vi "Autonomous Independent.vi"() -> ()   [LabVIEW 2016]
doc: "This VI is called when autonomous begins, and will automatically be terminated when autonomous ends. You can carry out timed or sensor driven robot movement independently without needing to return to the caller."
uses:
  <vilib>/Rock Robotics/WPI/Utilities/WPI_GetSetVariantRefNum.vi
  <vilib>/Rock Robotics/Network Tables/NT Write Numeric Array.vi
  Alliance_ID.vi
  <vilib>/Rock Robotics/WPI/RobotDrive/WPI_RobotDriveArcadeDrive_Standard(NoSaturation).vi
  <vilib>/Rock Robotics/Network Tables/NT Read String.vi
  <vilib>/Rock Robotics/Network Tables/NT Write Number.vi
panel:
  out "Completed Task 8":bool
  in  "Past the Peg. No Turn":i32=18
  out "Completed Task 7":bool
  in  "Ticks to the Peg 6":i32=3
  in  "Ticks to the Peg 5":i32=19
  out "Count":dbl
  in  "Ticks to the Peg 4":i32=3
  out "Completed Task 6":bool
  out "Completed Task 5":bool
  out "Completed Task 4":bool
  out "Completed Task 3":bool
  in  "Ticks to the Peg 3":i32=20
  out "Completed Task 1":bool
  in  "Ticks to the Peg 2":i32=15
  out "Left + Right OverSpeed":cluster{dbl, dbl}(knob)={10.0, -10.0} scale=-10.0..10.0
  out "Difference":dbl(knob) scale=0.0..50.0
  out "Right Wheel Sensor Count":dbl
  out "Left Wheel Sensor Count":dbl
  in  "Reset Counters":bool
  # "ALT 1"
  # "Position 3"
  # "16"
  # "20"
  # "Forward"
  # "3"
  # "Foward to the Left"
  # "4"
  # "Position 1"
  # "20"
  # "Forward"
  # "3"
  # "Foward to the Right"
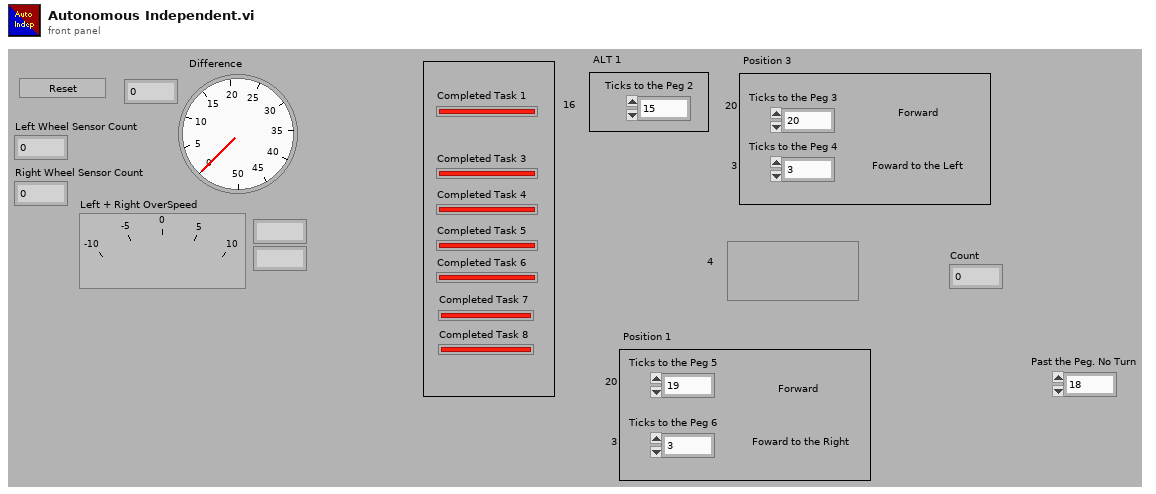
[diagram p1: front panel]
types:
  T1 = typedef "WPI_DriverStationPositionInfo.ctl" = enum16{"1", "2", "3"}
  T2 = typedef "WPI_DriverStationAllianceInfo.ctl" = enum16{"Red", "Blue", "Invalid"}
  T3 = typedef "WPI_JoystickDevRef.ctl" = cluster{"Device":T4}
  T4 = typedef "WPI_JoystickDeviceEnum.ctl" = enum16{"USB 0", "USB 1", "USB 2", "USB 3", "USB 4", "USB 5"}
  T5 = typedef "WPI_RobotDriveDevRef.ctl" = cluster{"DevStatus":errorcluster, "Motors[]":T6[], "Square Inputs":bool, "Max Output":dbl}
  T6 = typedef "WPI_MotorControlDeviceRef.ctl" = cluster{"DeviceStatus":errorcluster, "Type":T7, "PWM":cluster{"PWM Channel":T8, "DeadBand":T9}, "CAN":cluster{"Device Number":u8, "SetOutput VI Ref":variant, "GetOutput VI Ref":variant, "Enable VI Ref":variant, "Disable VI Ref":variant, "Data":variant}, "Invert":bool}
  T7 = typedef "WPI_MotorControlType.ctl" = enum16{"PWM", "CAN"}
  T8 = typedef "FPGA_DIOPWMChannel.ctl" = enum8{"PWM 0", "PWM 1", "PWM 2", "PWM 3", "PWM 4", "PWM 5", "PWM 6", "PWM 7", "PWM 8", "PWM 9", "PWM MXP 0", "PWM MXP 1", "PWM MXP 2", "PWM MXP 3", "PWM MXP 4", "PWM MXP 5", "PWM MXP 6", "PWM MXP 7", "PWM MXP 8", "PWM MXP 9", "Invalid"}
  T9 = typedef "WPI_PWMDeadband.ctl" = cluster{"Name":string, "maxPositivePwm":i32, "minPositivePwm":i32, "centerPwm":i32, "maxNegativePwm":i32, "minNegativePwm":i32, "angularRange":u16}
  T10 = typedef "WPI_CounterDevRef.ctl" = cluster{"DevStatus":errorcluster, "CntIndex":T11}
  T11 = typedef "FPGA_CounterCtrSystemIndex.ctl" = enum8{"Ctr 0", "Ctr 1", "Ctr 2", "Ctr 3", "Ctr 4", "Ctr 5", "Ctr 6", "Ctr 7", "Invalid"}
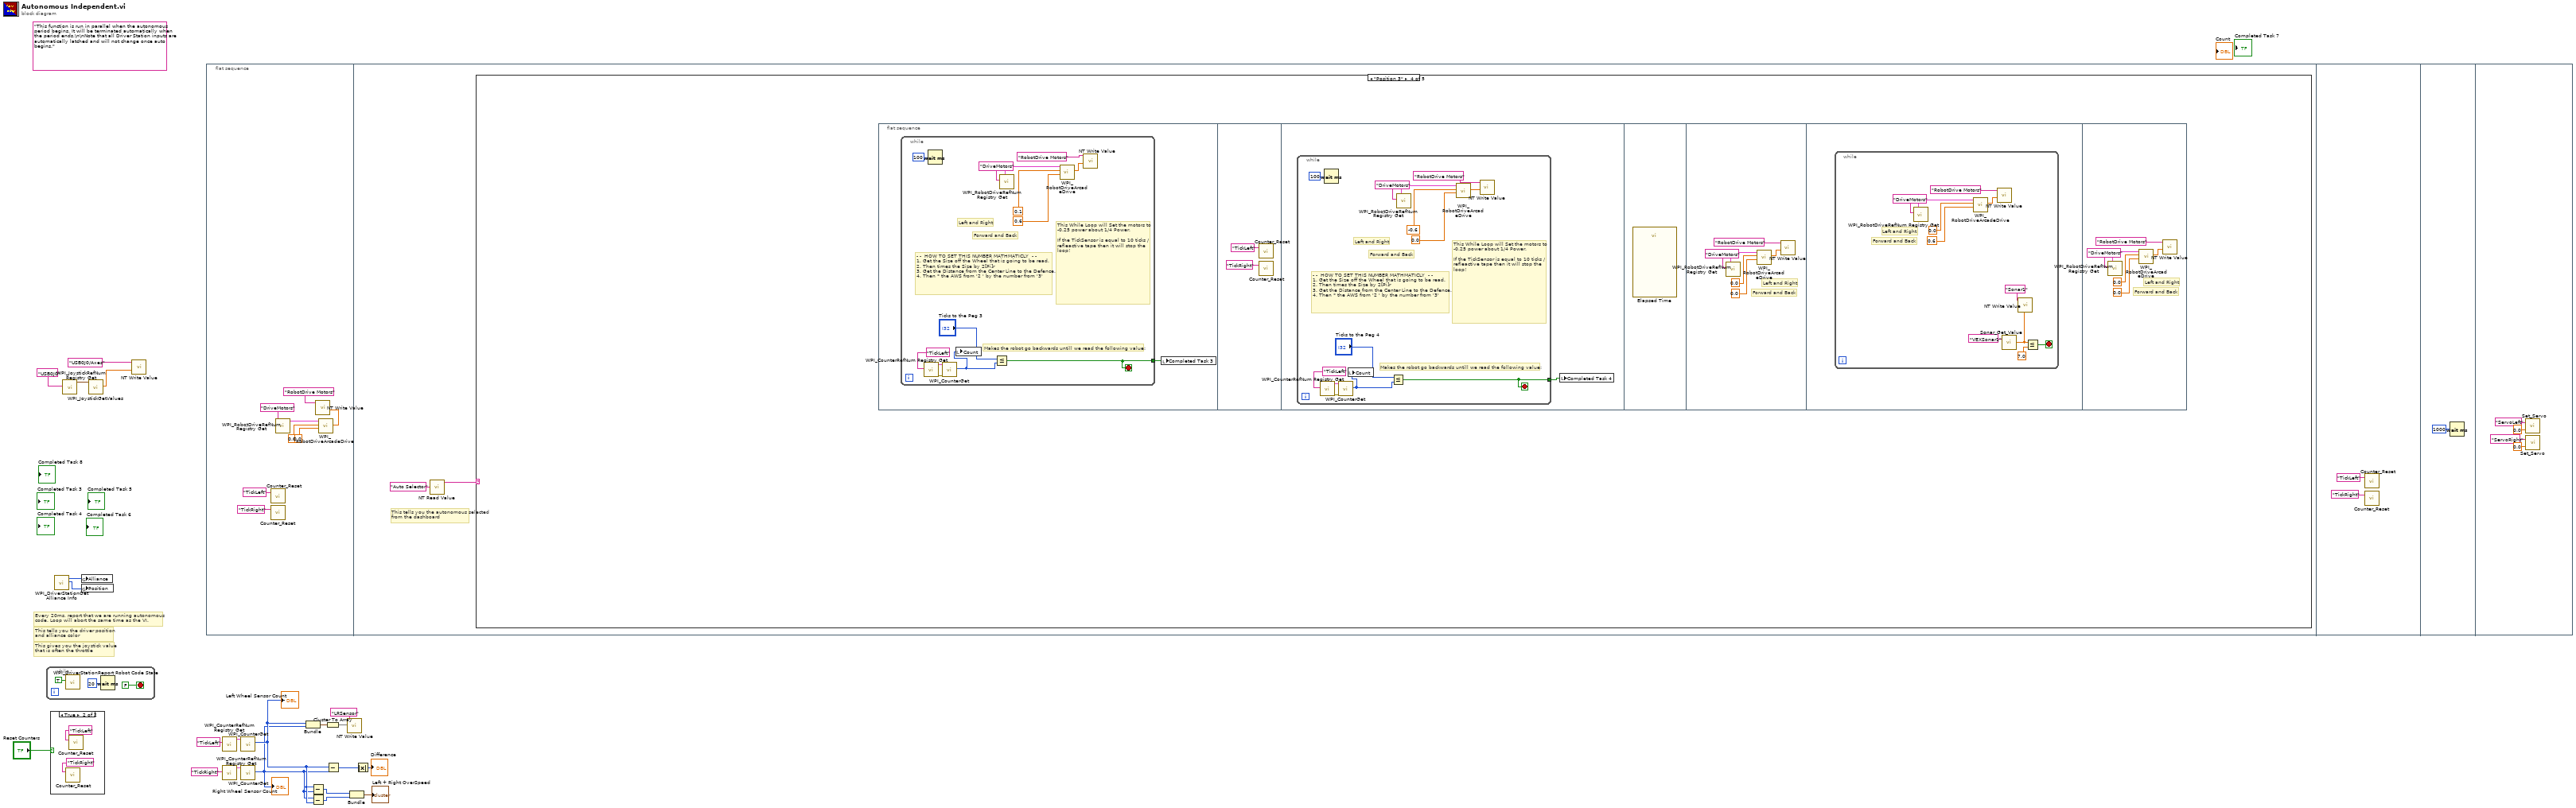
[diagram p0: block diagram]
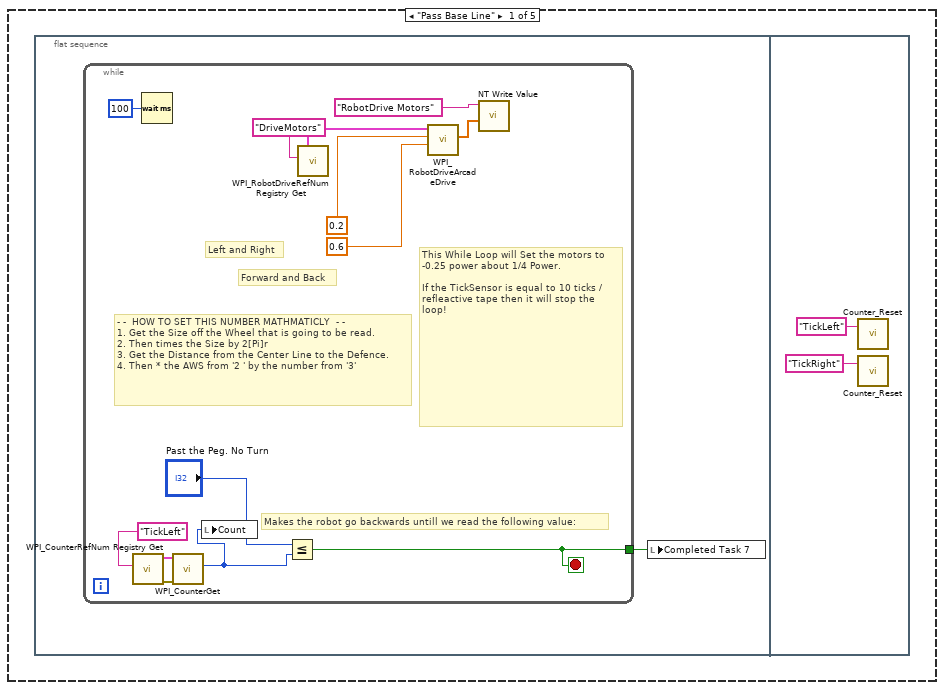
[diagram p2: hidden frame]
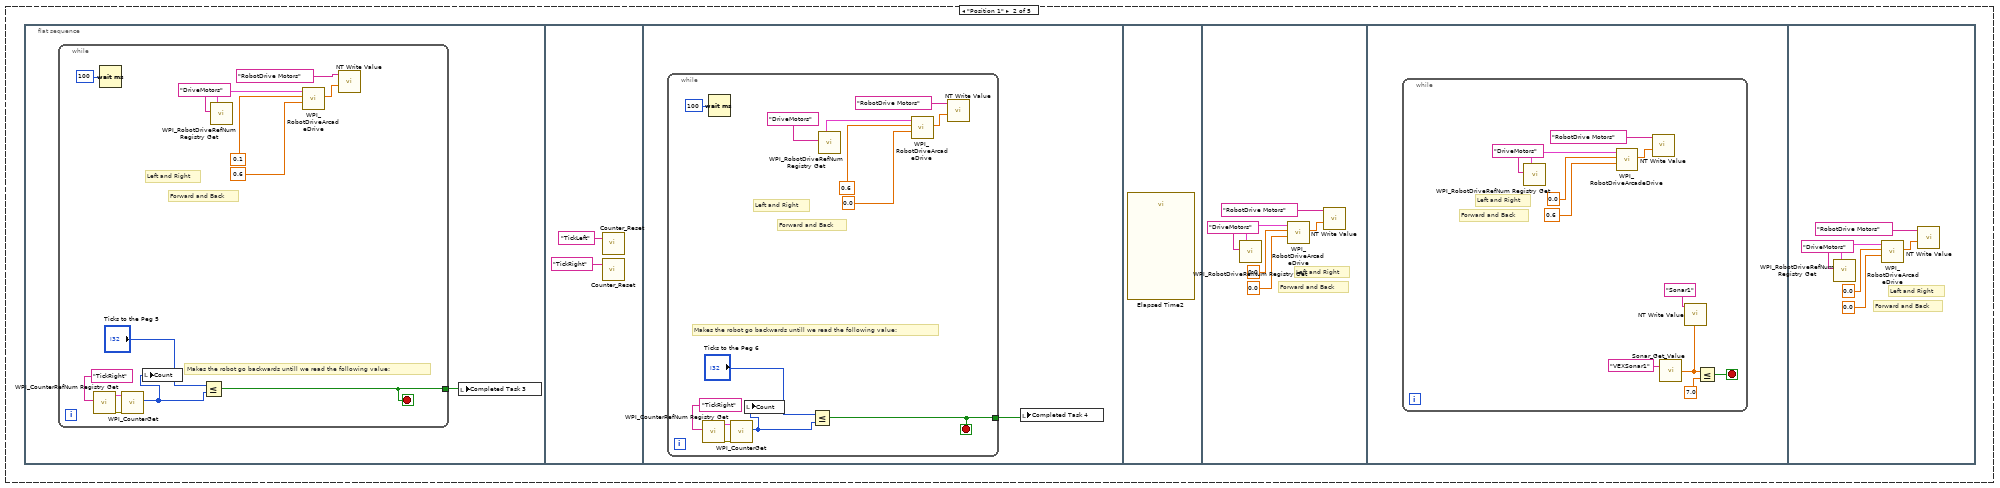
[diagram p3: hidden frame]
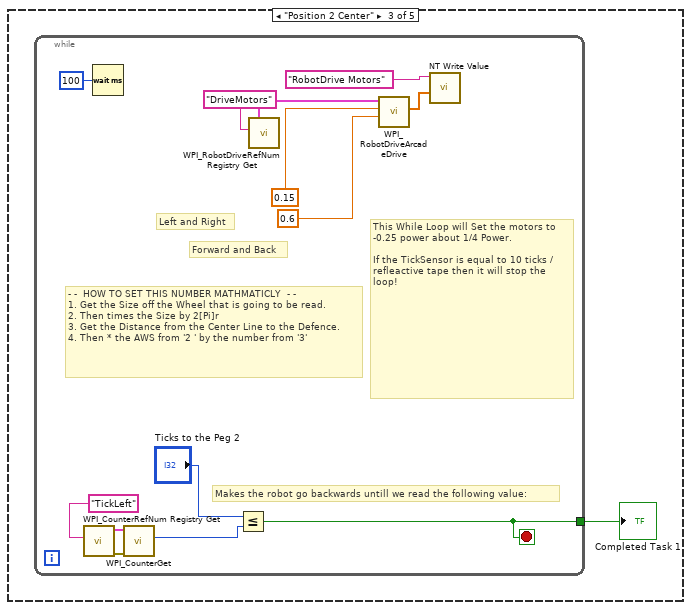
[diagram p4: hidden frame]
diagram:
  (unwired) "This function is run in parallel when the autonomous period begins. It will be terminated automatically when the period ends.\n\nNote that all Driver Station inputs are automatically latched and will not change once auto begins."
  # "Every 20ms, report that we are running autonomous\ncode. Loop will abort the same time as the VI."
  # "This gives you the joystick value\nthat is often the throttle"
  # "This tells you the driver position\nand alliance color"
  n1 = while {
    stop <- FALSE stop-if-true
    n2 = call <vilib>:"WPI_DriverStationReport Robot Code State.vi"("Autonomous"=TRUE) -> ()  [unwired: 10 in, 1 out]
    n3 = Wait (ms)(milliseconds to wait=u32 20) -> ()  [unwired: 1 out]
  }
  n4 = case shown="True" "Reset Counters" {
    frame False {
      # "Do nothing."
    }
    frame True {
      n5 = call "Counter_Reset.vi"("Control"="TickRight" ("refnum name")) -> ()  [unwired: 1 in, 2 out]
      n6 = call "Counter_Reset.vi"("Control"="TickLeft" ("refnum name")) -> ()  [unwired: 1 in, 2 out]
    }
  }
  n7 = call <vilib>:"WPI_DriverStationGet Alliance Info.vi"() -> ("Position"=w6:T1, "Alliance"=w7:T2)  [unwired: 10 out]
  n8 = call <vilib>:"WPI_JoystickRefNum Registry Get.vi"("refnum name"="USB0J0") -> ("JoystickDevRef"=w20:T3)  [unwired: 1 in, 9 out]
  n9 = global write "Alliance_ID.vi" "Alliance"(w7) -> ()
  n10 = global write "Alliance_ID.vi" "Position"(w6) -> ()
  n11 = call <vilib>:"WPI_JoystickGetValues.vi"("JoystickDevRef"=w20) -> ("Axes"=w18:dbl[])  [unwired: 6 in, 4 out]
  n12 = call-poly <vilib>:"NT Write Value.vi"("Numeric Array"=w18, "Name"="USB0J0/Axes") -> ()  [unwired: 9 in, 1 out]
  n13 = flat-sequence {
    frame #0 {
      n14 = call "Counter_Reset.vi"("Control"="TickLeft" ("refnum name")) -> ()  [unwired: 1 in, 2 out]
      n15 = call "Counter_Reset.vi"("Control"="TickRight" ("refnum name")) -> ()  [unwired: 1 in, 2 out]
      n16 = call <vilib>:"WPI_RobotDriveRefNum Registry Get.vi"("refnum name"="DriveMotors") -> ("RobotDriveDevRef"=w34:T5)  [unwired: 1 in, 9 out]
      n17 = call-poly <vilib>:"WPI_RobotDriveArcadeDrive.vi"("Y axis value"=0.0 ("X axis value"), "X axis value"=0.0, "RobotDriveDevRef"=w34) -> ("Motor Values"=w32:dbl[])  [unwired: 1 in, 7 out]
      n18 = call-poly <vilib>:"NT Write Value.vi"("Numeric Array"=w32, "Name"="RobotDrive Motors") -> ()  [unwired: 9 in, 1 out]
    }
    frame #1 {
      # "This tells you the autonomous selected\nfrom the dashboard"
      n19 = call-poly <vilib>:"NT Read Value.vi"("Name"="Auto Selector") -> ("String"=w35:string)  [unwired: 9 in, 1 out]
      n20 = case shown="\"Position 3\"" w35 {
        frame "Pass Base Line" {
          n21 = flat-sequence {
            frame #0 {
              n22 = while {
                tunnel: [w40] -> w37
                stop <- w40 stop-if-true
                # "- -  HOW TO SET THIS NUMBER MATHMATICLY  - - \n1. Get the Size off the Wheel that is going to be read.\n2. Then times the Size by 2[Pi]r\n3. Get the Distance from the Center Line to the Defence.\n4. Then * the AWS from '2 ' by the number from '3'"
                # "Makes the robot go backwards untill we read the following value:"
                # "This While Loop will Set the motors to -0.25 power about 1/4 Power.\n\nIf the TickSensor is equal to 10 ticks / refleactive tape then it will stop the loop!"
                # "Forward and Back"
                # "Left and Right"
                n23 = call <vilib>:"WPI_CounterRefNum Registry Get.vi"("refnum name"="TickLeft") -> ("error out"=w49:errorcluster, "CounterDevRef"=w48:T10)  [unwired: 9 in]
                n24 = Wait (ms)(milliseconds to wait=u32 100) -> ()  [unwired: 1 out]
                n25 = call <vilib>:"WPI_CounterGet.vi"("error in (no error)"=w49, "CounterDevRef in"=w48) -> ("Value"=w38:i32)  [unwired: 4 in, 5 out]
                n26 = local write "Count"(w38) -> ()
                n27 = Less Or Equal?(x="Past the Peg. No Turn", y=w38) -> (x <= y?=w40:bool)
                n28 = call <vilib>:"WPI_RobotDriveRefNum Registry Get.vi"("refnum name"="DriveMotors") -> ("RobotDriveDevRef"=w47:T5)  [unwired: 1 in, 9 out]
                n29 = call-poly <vilib>:"WPI_RobotDriveArcadeDrive.vi"("Y axis value"=0.6 ("X axis value"), "X axis value"=0.2, "RobotDriveDevRef"=w47) -> ("Motor Values"=w45:dbl[])  [unwired: 1 in, 7 out]
                n30 = call-poly <vilib>:"NT Write Value.vi"("Numeric Array"=w45, "Name"="RobotDrive Motors") -> ()  [unwired: 9 in, 1 out]
              }
              n31 = local write "Completed Task 7"(w37) -> ()
            }
            frame #1 {
              n32 = call "Counter_Reset.vi"("Control"="TickLeft" ("refnum name")) -> ()  [unwired: 1 in, 2 out]
              n33 = call "Counter_Reset.vi"("Control"="TickRight" ("refnum name")) -> ()  [unwired: 1 in, 2 out]
            }
          }
        }
        frame "Position 1" {
          n34 = flat-sequence {
            frame #0 {
              n35 = while {
                tunnel: [w56] -> w53
                stop <- w56 stop-if-true
                # "Makes the robot go backwards untill we read the following value:"
                # "Forward and Back"
                # "Left and Right"
                n36 = call <vilib>:"WPI_CounterRefNum Registry Get.vi"("refnum name"="TickRight") -> ("error out"=w65:errorcluster, "CounterDevRef"=w64:T10)  [unwired: 9 in]
                n37 = Wait (ms)(milliseconds to wait=u32 100) -> ()  [unwired: 1 out]
                n38 = call <vilib>:"WPI_CounterGet.vi"("error in (no error)"=w65, "CounterDevRef in"=w64) -> ("Value"=w55:i32)  [unwired: 4 in, 5 out]
                n39 = local write "Count"(w55) -> ()
                n40 = Less Or Equal?(x="Ticks to the Peg 5", y=w55) -> (x <= y?=w56:bool)
                n41 = call <vilib>:"WPI_RobotDriveRefNum Registry Get.vi"("refnum name"="DriveMotors") -> ("RobotDriveDevRef"=w63:T5)  [unwired: 1 in, 9 out]
                n42 = call-poly <vilib>:"WPI_RobotDriveArcadeDrive.vi"("Y axis value"=0.6 ("X axis value"), "X axis value"=0.1, "RobotDriveDevRef"=w63) -> ("Motor Values"=w61:dbl[])  [unwired: 1 in, 7 out]
                n43 = call-poly <vilib>:"NT Write Value.vi"("Numeric Array"=w61, "Name"="RobotDrive Motors") -> ()  [unwired: 9 in, 1 out]
              }
              n44 = local write "Completed Task 3"(w53) -> ()
            }
            frame #1 {
              n45 = call "Counter_Reset.vi"("Control"="TickLeft" ("refnum name")) -> ()  [unwired: 1 in, 2 out]
              n46 = call "Counter_Reset.vi"("Control"="TickRight" ("refnum name")) -> ()  [unwired: 1 in, 2 out]
            }
            frame #2 {
              n47 = while {
                tunnel: [w72] -> w69
                stop <- w72 stop-if-true
                # "Makes the robot go backwards untill we read the following value:"
                # "Forward and Back"
                # "Left and Right"
                n48 = call <vilib>:"WPI_CounterRefNum Registry Get.vi"("refnum name"="TickRight") -> ("error out"=w81:errorcluster, "CounterDevRef"=w80:T10)  [unwired: 9 in]
                n49 = Wait (ms)(milliseconds to wait=u32 100) -> ()  [unwired: 1 out]
                n50 = call <vilib>:"WPI_CounterGet.vi"("error in (no error)"=w81, "CounterDevRef in"=w80) -> ("Value"=w71:i32)  [unwired: 4 in, 5 out]
                n51 = local write "Count"(w71) -> ()
                n52 = Less Or Equal?(x="Ticks to the Peg 6", y=w71) -> (x <= y?=w72:bool)
                n53 = call <vilib>:"WPI_RobotDriveRefNum Registry Get.vi"("refnum name"="DriveMotors") -> ("RobotDriveDevRef"=w79:T5)  [unwired: 1 in, 9 out]
                n54 = call-poly <vilib>:"WPI_RobotDriveArcadeDrive.vi"("Y axis value"=0.0 ("X axis value"), "X axis value"=0.6, "RobotDriveDevRef"=w79) -> ("Motor Values"=w77:dbl[])  [unwired: 1 in, 7 out]
                n55 = call-poly <vilib>:"NT Write Value.vi"("Numeric Array"=w77, "Name"="RobotDrive Motors") -> ()  [unwired: 9 in, 1 out]
              }
              n56 = local write "Completed Task 4"(w69) -> ()
            }
            frame #3 {
              n57 = call "Elapsed Time2"() -> ()  [unwired: 12 in, 8 out]
            }
            frame #4 {
              # "Forward and Back"
              # "Left and Right"
              n58 = call <vilib>:"WPI_RobotDriveRefNum Registry Get.vi"("refnum name"="DriveMotors") -> ("RobotDriveDevRef"=w88:T5)  [unwired: 1 in, 9 out]
              n59 = call-poly <vilib>:"WPI_RobotDriveArcadeDrive.vi"("Y axis value"=0.0 ("X axis value"), "X axis value"=0.0, "RobotDriveDevRef"=w88) -> ("Motor Values"=w86:dbl[])  [unwired: 1 in, 7 out]
              n60 = call-poly <vilib>:"NT Write Value.vi"("Numeric Array"=w86, "Name"="RobotDrive Motors") -> ()  [unwired: 9 in, 1 out]
            }
            frame #5 {
              n61 = while {
                stop <- w98 stop-if-true
                # "Forward and Back"
                # "Left and Right"
                n62 = call <vilib>:"WPI_RobotDriveRefNum Registry Get.vi"("refnum name"="DriveMotors") -> ("RobotDriveDevRef"=w96:T5)  [unwired: 1 in, 9 out]
                n63 = call-poly <vilib>:"WPI_RobotDriveArcadeDrive.vi"("Y axis value"=0.6 ("X axis value"), "X axis value"=0.0, "RobotDriveDevRef"=w96) -> ("Motor Values"=w94:dbl[])  [unwired: 1 in, 7 out]
                n64 = call-poly <vilib>:"NT Write Value.vi"("Numeric Array"=w94, "Name"="RobotDrive Motors") -> ()  [unwired: 9 in, 1 out]
                n65 = call "Sonar_Get_Value.vi"("RefName"="VEXSonar1") -> ("Inches Out"=w89:dbl)  [unwired: 1 in, 2 out]
                n66 = call-poly <vilib>:"NT Write Value.vi"("Numeric"=w89, "Name"="Sonar1") -> ()  [unwired: 9 in, 1 out]
                n67 = Less Or Equal?(x=w89, y=7.0) -> (x <= y?=w98:bool)
              }
            }
            frame #6 {
              # "Forward and Back"
              # "Left and Right"
              n68 = call <vilib>:"WPI_RobotDriveRefNum Registry Get.vi"("refnum name"="DriveMotors") -> ("RobotDriveDevRef"=w105:T5)  [unwired: 1 in, 9 out]
              n69 = call-poly <vilib>:"WPI_RobotDriveArcadeDrive.vi"("Y axis value"=0.0 ("X axis value"), "X axis value"=0.0, "RobotDriveDevRef"=w105) -> ("Motor Values"=w103:dbl[])  [unwired: 1 in, 7 out]
              n70 = call-poly <vilib>:"NT Write Value.vi"("Numeric Array"=w103, "Name"="RobotDrive Motors") -> ()  [unwired: 9 in, 1 out]
            }
          }
        }
        frame "Position 2 Center" {
          n71 = while {
            tunnel: [w107] -> w106
            stop <- w107 stop-if-true
            # "- -  HOW TO SET THIS NUMBER MATHMATICLY  - - \n1. Get the Size off the Wheel that is going to be read.\n2. Then times the Size by 2[Pi]r\n3. Get the Distance from the Center Line to the Defence.\n4. Then * the AWS from '2 ' by the number from '3'"
            # "Makes the robot go backwards untill we read the following value:"
            # "This While Loop will Set the motors to -0.25 power about 1/4 Power.\n\nIf the TickSensor is equal to 10 ticks / refleactive tape then it will stop the loop!"
            # "Forward and Back"
            # "Left and Right"
            n72 = call <vilib>:"WPI_CounterRefNum Registry Get.vi"("refnum name"="TickLeft") -> ("error out"=w118:errorcluster, "CounterDevRef"=w117:T10)  [unwired: 9 in]
            n73 = Wait (ms)(milliseconds to wait=u32 100) -> ()  [unwired: 1 out]
            n74 = call <vilib>:"WPI_CounterGet.vi"("error in (no error)"=w118, "CounterDevRef in"=w117) -> ("Value"=w109:i32)  [unwired: 4 in, 5 out]
            n75 = Less Or Equal?(x="Ticks to the Peg 2", y=w109) -> (x <= y?=w107:bool)
            n76 = call <vilib>:"WPI_RobotDriveRefNum Registry Get.vi"("refnum name"="DriveMotors") -> ("RobotDriveDevRef"=w116:T5)  [unwired: 1 in, 9 out]
            n77 = call-poly <vilib>:"WPI_RobotDriveArcadeDrive.vi"("Y axis value"=0.6 ("X axis value"), "X axis value"=0.15, "RobotDriveDevRef"=w116) -> ("Motor Values"=w114:dbl[])  [unwired: 1 in, 7 out]
            n78 = call-poly <vilib>:"NT Write Value.vi"("Numeric Array"=w114, "Name"="RobotDrive Motors") -> ()  [unwired: 9 in, 1 out]
          }
          "Completed Task 1" <- w106
        }
        frame "Position 3" {
          n79 = flat-sequence {
            frame #0 {
              n80 = while {
                tunnel: [w123] -> w120
                stop <- w123 stop-if-true
                # "- -  HOW TO SET THIS NUMBER MATHMATICLY  - - \n1. Get the Size off the Wheel that is going to be read.\n2. Then times the Size by 2[Pi]r\n3. Get the Distance from the Center Line to the Defence.\n4. Then * the AWS from '2 ' by the number from '3'"
                # "Makes the robot go backwards untill we read the following value:"
                # "This While Loop will Set the motors to -0.25 power about 1/4 Power.\n\nIf the TickSensor is equal to 10 ticks / refleactive tape then it will stop the loop!"
                # "Forward and Back"
                # "Left and Right"
                n81 = call <vilib>:"WPI_CounterRefNum Registry Get.vi"("refnum name"="TickLeft") -> ("error out"=w132:errorcluster, "CounterDevRef"=w131:T10)  [unwired: 9 in]
                n82 = Wait (ms)(milliseconds to wait=u32 100) -> ()  [unwired: 1 out]
                n83 = call <vilib>:"WPI_CounterGet.vi"("error in (no error)"=w132, "CounterDevRef in"=w131) -> ("Value"=w121:i32)  [unwired: 4 in, 5 out]
                n84 = local write "Count"(w121) -> ()
                n85 = Less Or Equal?(x="Ticks to the Peg 3", y=w121) -> (x <= y?=w123:bool)
                n86 = call <vilib>:"WPI_RobotDriveRefNum Registry Get.vi"("refnum name"="DriveMotors") -> ("RobotDriveDevRef"=w130:T5)  [unwired: 1 in, 9 out]
                n87 = call-poly <vilib>:"WPI_RobotDriveArcadeDrive.vi"("Y axis value"=0.6 ("X axis value"), "X axis value"=0.1, "RobotDriveDevRef"=w130) -> ("Motor Values"=w128:dbl[])  [unwired: 1 in, 7 out]
                n88 = call-poly <vilib>:"NT Write Value.vi"("Numeric Array"=w128, "Name"="RobotDrive Motors") -> ()  [unwired: 9 in, 1 out]
              }
              n89 = local write "Completed Task 3"(w120) -> ()
            }
            frame #1 {
              n90 = call "Counter_Reset.vi"("Control"="TickLeft" ("refnum name")) -> ()  [unwired: 1 in, 2 out]
              n91 = call "Counter_Reset.vi"("Control"="TickRight" ("refnum name")) -> ()  [unwired: 1 in, 2 out]
            }
            frame #2 {
              n92 = while {
                tunnel: [w139] -> w136
                stop <- w139 stop-if-true
                # "- -  HOW TO SET THIS NUMBER MATHMATICLY  - - \n1. Get the Size off the Wheel that is going to be read.\n2. Then times the Size by 2[Pi]r\n3. Get the Distance from the Center Line to the Defence.\n4. Then * the AWS from '2 ' by the number from '3'"
                # "Makes the robot go backwards untill we read the following value:"
                # "This While Loop will Set the motors to -0.25 power about 1/4 Power.\n\nIf the TickSensor is equal to 10 ticks / refleactive tape then it will stop the loop!"
                # "Forward and Back"
                # "Left and Right"
                n93 = call <vilib>:"WPI_CounterRefNum Registry Get.vi"("refnum name"="TickLeft") -> ("error out"=w148:errorcluster, "CounterDevRef"=w147:T10)  [unwired: 9 in]
                n94 = Wait (ms)(milliseconds to wait=u32 100) -> ()  [unwired: 1 out]
                n95 = call <vilib>:"WPI_CounterGet.vi"("error in (no error)"=w148, "CounterDevRef in"=w147) -> ("Value"=w137:i32)  [unwired: 4 in, 5 out]
                n96 = local write "Count"(w137) -> ()
                n97 = Less Or Equal?(x="Ticks to the Peg 4", y=w137) -> (x <= y?=w139:bool)
                n98 = call <vilib>:"WPI_RobotDriveRefNum Registry Get.vi"("refnum name"="DriveMotors") -> ("RobotDriveDevRef"=w146:T5)  [unwired: 1 in, 9 out]
                n99 = call-poly <vilib>:"WPI_RobotDriveArcadeDrive.vi"("Y axis value"=0.0 ("X axis value"), "X axis value"=-0.6, "RobotDriveDevRef"=w146) -> ("Motor Values"=w144:dbl[])  [unwired: 1 in, 7 out]
                n100 = call-poly <vilib>:"NT Write Value.vi"("Numeric Array"=w144, "Name"="RobotDrive Motors") -> ()  [unwired: 9 in, 1 out]
              }
              n101 = local write "Completed Task 4"(w136) -> ()
            }
            frame #3 {
              n102 = call "Elapsed Time"() -> ()  [unwired: 12 in, 8 out]
            }
            frame #4 {
              # "Forward and Back"
              # "Left and Right"
              n103 = call <vilib>:"WPI_RobotDriveRefNum Registry Get.vi"("refnum name"="DriveMotors") -> ("RobotDriveDevRef"=w155:T5)  [unwired: 1 in, 9 out]
              n104 = call-poly <vilib>:"WPI_RobotDriveArcadeDrive.vi"("Y axis value"=0.0 ("X axis value"), "X axis value"=0.0, "RobotDriveDevRef"=w155) -> ("Motor Values"=w153:dbl[])  [unwired: 1 in, 7 out]
              n105 = call-poly <vilib>:"NT Write Value.vi"("Numeric Array"=w153, "Name"="RobotDrive Motors") -> ()  [unwired: 9 in, 1 out]
            }
            frame #5 {
              n106 = while {
                stop <- w165 stop-if-true
                # "Forward and Back"
                # "Left and Right"
                n107 = call <vilib>:"WPI_RobotDriveRefNum Registry Get.vi"("refnum name"="DriveMotors") -> ("RobotDriveDevRef"=w163:T5)  [unwired: 1 in, 9 out]
                n108 = call-poly <vilib>:"WPI_RobotDriveArcadeDrive.vi"("Y axis value"=0.6 ("X axis value"), "X axis value"=0.0, "RobotDriveDevRef"=w163) -> ("Motor Values"=w161:dbl[])  [unwired: 1 in, 7 out]
                n109 = call-poly <vilib>:"NT Write Value.vi"("Numeric Array"=w161, "Name"="RobotDrive Motors") -> ()  [unwired: 9 in, 1 out]
                n110 = call "Sonar_Get_Value.vi"("RefName"="VEXSonar1") -> ("Inches Out"=w156:dbl)  [unwired: 1 in, 2 out]
                n111 = call-poly <vilib>:"NT Write Value.vi"("Numeric"=w156, "Name"="Sonar1") -> ()  [unwired: 9 in, 1 out]
                n112 = Less Or Equal?(x=w156, y=7.0) -> (x <= y?=w165:bool)
              }
            }
            frame #6 {
              # "Forward and Back"
              # "Left and Right"
              n113 = call <vilib>:"WPI_RobotDriveRefNum Registry Get.vi"("refnum name"="DriveMotors") -> ("RobotDriveDevRef"=w172:T5)  [unwired: 1 in, 9 out]
              n114 = call-poly <vilib>:"WPI_RobotDriveArcadeDrive.vi"("Y axis value"=0.0 ("X axis value"), "X axis value"=0.0, "RobotDriveDevRef"=w172) -> ("Motor Values"=w170:dbl[])  [unwired: 1 in, 7 out]
              n115 = call-poly <vilib>:"NT Write Value.vi"("Numeric Array"=w170, "Name"="RobotDrive Motors") -> ()  [unwired: 9 in, 1 out]
            }
          }
        }
        frame "0", "DefaultCode", "None", Default {
          # "You can put your main auto here, or you can right-click on the case and make any\nother frame be the default case."
          # "This is the frame that will execute if no selection is made, or if it is not recognized"
        }
      }
    }
    frame #2 {
      n116 = call "Counter_Reset.vi"("Control"="TickLeft" ("refnum name")) -> ()  [unwired: 1 in, 2 out]
      n117 = call "Counter_Reset.vi"("Control"="TickRight" ("refnum name")) -> ()  [unwired: 1 in, 2 out]
    }
    frame #3 {
      n118 = Wait (ms)(milliseconds to wait=u32 1000) -> ()  [unwired: 1 out]
    }
    frame #4 {
      n119 = call "Set_Servo.vi"("Set To"=0.0, "Servo To Control"="ServoLeft") -> ()  [unwired: 1 out]
      n120 = call "Set_Servo.vi"("Set To"=0.0, "Servo To Control"="ServoRight") -> ()  [unwired: 1 out]
    }
  }
  n121 = call <vilib>:"WPI_CounterRefNum Registry Get.vi"("refnum name"="TickLeft") -> ("CounterDevRef"=w15:T10)  [unwired: 9 in, 1 out]
  n122 = call <vilib>:"WPI_CounterRefNum Registry Get.vi"("refnum name"="TickRight") -> ("CounterDevRef"=w14:T10)  [unwired: 9 in, 1 out]
  n123 = call <vilib>:"WPI_CounterGet.vi"("CounterDevRef in"=w15) -> ("Value"=w3:i32)  [unwired: 5 in, 5 out]
  "Left Wheel Sensor Count" <- w3
  n124 = call <vilib>:"WPI_CounterGet.vi"("CounterDevRef in"=w14) -> ("Value"=w2:i32)  [unwired: 5 in, 5 out]
  "Right Wheel Sensor Count" <- w2
  n125 = Bundle("Value"=w3, "Value"=w2) -> (w5:cluster{"Value":i32, "Value":i32})  [unwired: 1 in]
  n126 = Subtract(x=w3, y=w2) -> (x-y=w10:i32)
  n127 = Subtract(x=w2, y=w3) -> (x-y=w9:i32)
  n128 = Cluster To Array(cluster=w5) -> (array=w4:i32[])
  n129 = Subtract(x=w3, y=w2) -> (x-y=w13:i32)
  n130 = call-poly <vilib>:"NT Write Value.vi"("Numeric Array"=w4, "Name"="LRSensor") -> ()  [unwired: 9 in, 1 out]
  n131 = Bundle(w10, w9) -> (→"Left + Right OverSpeed":cluster{i32, i32})  [unwired: 1 in]
  n132 = Absolute Value(x=w13) -> (abs(x)=→"Difference":i32)
